vi "GenerateMapGraph.vi"() -> ()   [LabVIEW 2015]
panel:
  out "Numeric 1":i32
  out "Numeric 2":i32
  in  "Graph Parameters":T1={"Y_max"=10.0, "Y_min"=0.0, "X_max"=10.0, "X_min"=0.0}
  out "Output":cluster{dbl[], dbl[]}[](graph)
  in  "Input M":dbl[][](array[numeric])=[[14.0, 12.0, 6.0, 12.0], [10.0, 11.0, 10.0, 10.0], [8.0, 6.0, 10.0, 10.0], [10.0, 9.0, 1.0, 3.0], [0.0, 13.0, 1.0, 7.0]]
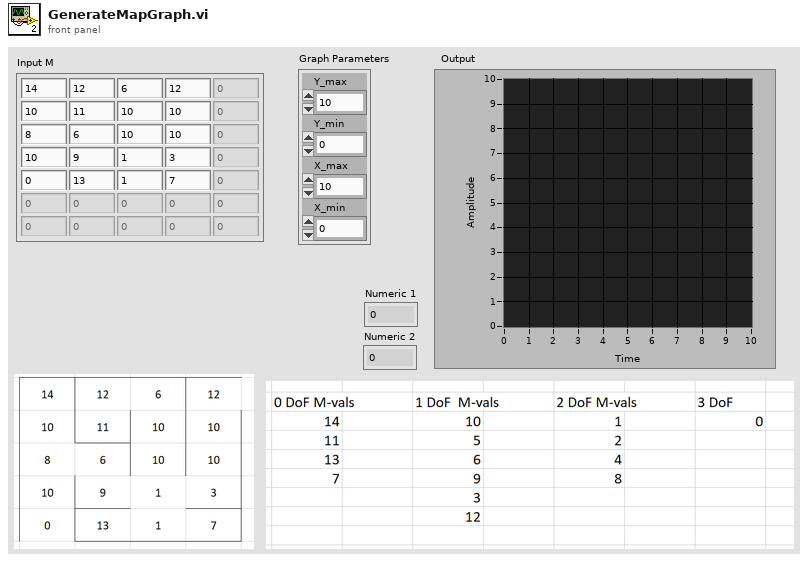
[diagram p1: front panel]
types:
  T1 = cluster{"Y_max":dbl, "Y_min":dbl, "X_max":dbl, "X_min":dbl}
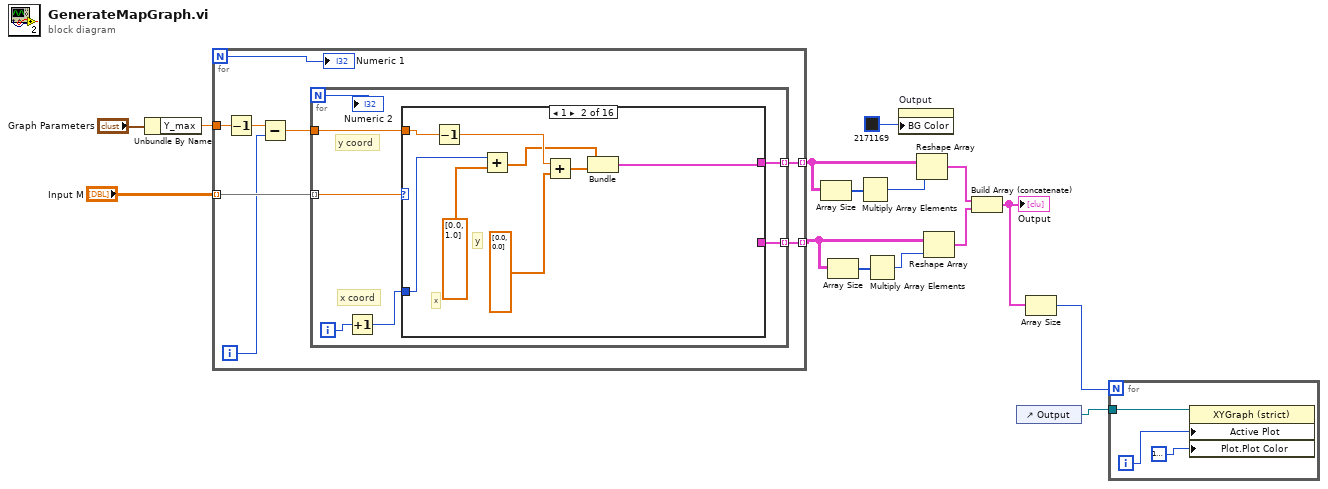
[diagram p0: block diagram]
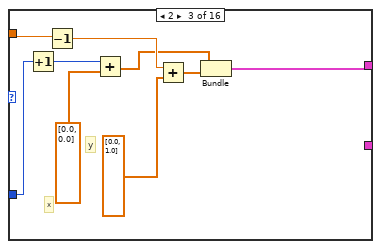
[diagram p3: hidden frame]
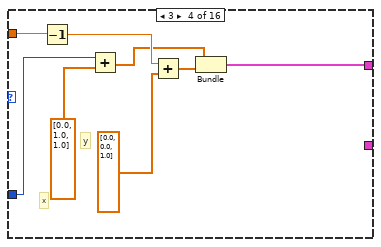
[diagram p4: hidden frame]
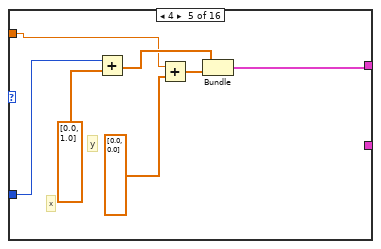
[diagram p5: hidden frame]
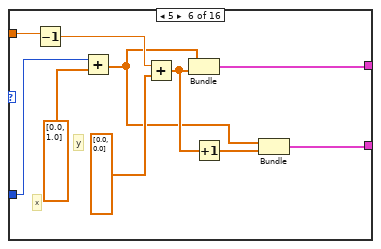
[diagram p6: hidden frame]
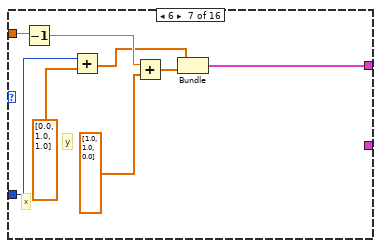
[diagram p7: hidden frame]
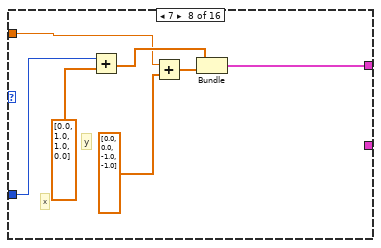
[diagram p8: hidden frame]
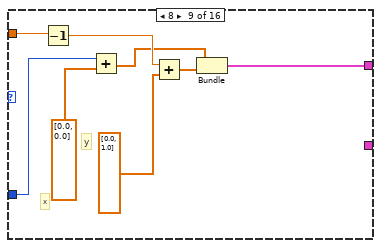
[diagram p9: hidden frame]
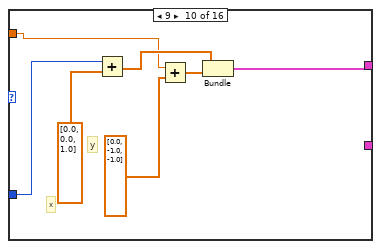
[diagram p10: hidden frame]
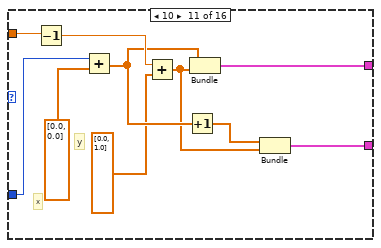
[diagram p11: hidden frame]
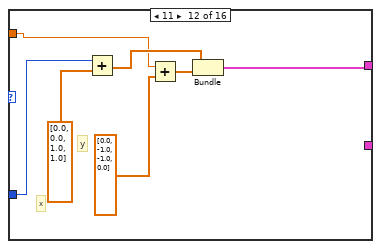
[diagram p12: hidden frame]
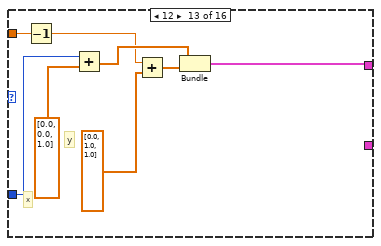
[diagram p13: hidden frame]
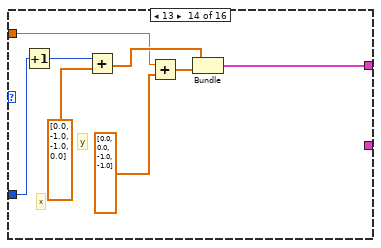
[diagram p14: hidden frame]
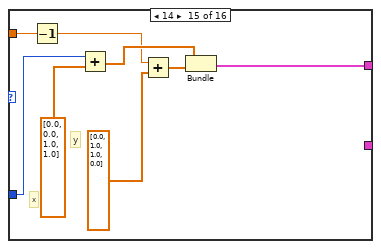
[diagram p15: hidden frame]
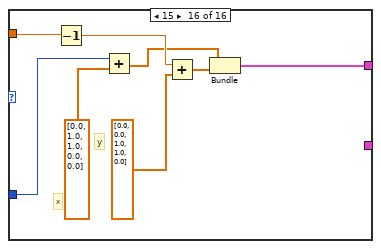
[diagram p16: hidden frame]
diagram:
  n1 = Unbundle By Name("Graph Parameters") -> ("Y_max"=w13:dbl)
  n2 = for {
    N -> [w21]
    tunnel: "Input M" -> [w23] mode=indexing
    tunnel: w13 -> [w22]
    tunnel: [w17] -> w12 mode=indexing
    tunnel: [w16] -> w5 mode=indexing
    i -> [w19]
    n3 = Decrement(x=w22) -> (x-1=w20:dbl)
    n4 = Subtract(x=w20, y=w19) -> (x-y=w18:dbl)
    n5 = for {
      N -> [w29]
      tunnel: w23 -> [w30] mode=indexing
      tunnel: w18 -> [w28]
      tunnel: [w25] -> w17 mode=indexing
      tunnel: [w24] -> w16 mode=indexing
      i -> [w27]
      # "x coord"
      # "y coord"
      n6 = Increment(x=w27) -> (x+1=w26:i32)
      n7 = case shown="1" w30 {
        tunnel: w28 -> [_ w32 w40 w49 w57 w67 w74 w81 w90 w98 w111 w113 w120 w129 w141 w146]
        tunnel: w26 -> [_ w31 w41 w50 w56 w68 w75 w82 w88 w96 w109 w115 w122 w130 w142 w145]
        tunnel: [_ w33 w39 w48 w58 w64 w73 w83 w89 w97 w110 w114 w121 w131 w137 w144] -> w25
        tunnel: [_ _ _ _ _ w63 _ _ _ _ w106 _ _ _ _ _] -> w24
        frame 0, Default {
        }
        frame 1 {
          # "y"
          # "x"
          n8 = Decrement(x=w32) -> (x-1=w38:dbl)
          n9 = Add(x=w31, y=dbl[] [0.0, 1.0] ("appended array")) -> (x+y=w37:dbl[])
          n10 = Add(x=w38, y=dbl[] [0.0, 0.0] ("appended array")) -> (x+y=w36:dbl[])
          n11 = Bundle(w37, w36) -> (w33:cluster{dbl[], dbl[]})  [unwired: 1 in]
        }
        frame 2 {
          # "y"
          # "x"
          n12 = Increment(x=w41) -> (x+1=w42:i32)
          n13 = Decrement(x=w40) -> (x-1=w47:dbl)
          n14 = Add(x=w42, y=dbl[] [0.0, 0.0] ("appended array")) -> (x+y=w46:dbl[])
          n15 = Add(x=w47, y=dbl[] [0.0, 1.0] ("appended array")) -> (x+y=w45:dbl[])
          n16 = Bundle(w46, w45) -> (w39:cluster{dbl[], dbl[]})  [unwired: 1 in]
        }
        frame 3 {
          # "y"
          # "x"
          n17 = Decrement(x=w49) -> (x-1=w55:dbl)
          n18 = Add(x=w50, y=dbl[] [0.0, 1.0, 1.0] ("appended array")) -> (x+y=w54:dbl[])
          n19 = Add(x=w55, y=dbl[] [0.0, 0.0, 1.0] ("appended array")) -> (x+y=w53:dbl[])
          n20 = Bundle(w54, w53) -> (w48:cluster{dbl[], dbl[]})  [unwired: 1 in]
        }
        frame 4 {
          # "y"
          # "x"
          n21 = Add(x=w56, y=dbl[] [0.0, 1.0] ("appended array")) -> (x+y=w62:dbl[])
          n22 = Add(x=w57, y=dbl[] [0.0, 0.0] ("appended array")) -> (x+y=w61:dbl[])
          n23 = Bundle(w62, w61) -> (w58:cluster{dbl[], dbl[]})  [unwired: 1 in]
        }
        frame 5 {
          # "y"
          # "x"
          n24 = Decrement(x=w67) -> (x-1=w69:dbl)
          n25 = Add(x=w68, y=dbl[] [0.0, 1.0] ("appended array")) -> (x+y=w66:dbl[])
          n26 = Add(x=w69, y=dbl[] [0.0, 0.0] ("appended array")) -> (x+y=w72:dbl[])
          n27 = Bundle(w66, w72) -> (w64:cluster{dbl[], dbl[]})  [unwired: 1 in]
          n28 = Increment(x=w72) -> (x+1=w65:dbl[])
          n29 = Bundle(w66, w65) -> (w63:cluster{dbl[], dbl[]})  [unwired: 1 in]
        }
        frame 6 {
          # "y"
          # "x"
          n30 = Decrement(x=w74) -> (x-1=w80:dbl)
          n31 = Add(x=w75, y=dbl[] [0.0, 1.0, 1.0] ("appended array")) -> (x+y=w79:dbl[])
          n32 = Add(x=w80, y=dbl[] [1.0, 1.0, 0.0] ("appended array")) -> (x+y=w78:dbl[])
          n33 = Bundle(w79, w78) -> (w73:cluster{dbl[], dbl[]})  [unwired: 1 in]
        }
        frame 7 {
          # "y"
          # "x"
          n34 = Add(x=w82, y=dbl[] [0.0, 1.0, 1.0, 0.0] ("appended array")) -> (x+y=w87:dbl[])
          n35 = Add(x=w81, y=dbl[] [0.0, 0.0, -1.0, -1.0] ("appended array")) -> (x+y=w86:dbl[])
          n36 = Bundle(w87, w86) -> (w83:cluster{dbl[], dbl[]})  [unwired: 1 in]
        }
        frame 8 {
          # "y"
          # "x"
          n37 = Decrement(x=w90) -> (x-1=w95:dbl)
          n38 = Add(x=w88, y=dbl[] [0.0, 0.0] ("appended array")) -> (x+y=w94:dbl[])
          n39 = Add(x=w95, y=dbl[] [0.0, 1.0] ("appended array")) -> (x+y=w93:dbl[])
          n40 = Bundle(w94, w93) -> (w89:cluster{dbl[], dbl[]})  [unwired: 1 in]
        }
        frame 9 {
          # "y"
          # "x"
          n41 = Add(x=w96, y=dbl[] [0.0, 0.0, 1.0] ("appended array")) -> (x+y=w102:dbl[])
          n42 = Add(x=w98, y=dbl[] [0.0, -1.0, -1.0] ("appended array")) -> (x+y=w101:dbl[])
          n43 = Bundle(w102, w101) -> (w97:cluster{dbl[], dbl[]})  [unwired: 1 in]
        }
        frame 10 {
          # "y"
          # "x"
          n44 = Decrement(x=w111) -> (x-1=w112:dbl)
          n45 = Add(x=w109, y=dbl[] [0.0, 0.0] ("appended array")) -> (x+y=w105:dbl[])
          n46 = Add(x=w112, y=dbl[] [0.0, 1.0] ("appended array")) -> (x+y=w103:dbl[])
          n47 = Increment(x=w105) -> (x+1=w107:dbl[])
          n48 = Bundle(w105, w103) -> (w110:cluster{dbl[], dbl[]})  [unwired: 1 in]
          n49 = Bundle(w107, w103) -> (w106:cluster{dbl[], dbl[]})  [unwired: 1 in]
        }
        frame 11 {
          # "y"
          # "x"
          n50 = Add(x=w115, y=dbl[] [0.0, 0.0, 1.0, 1.0] ("appended array")) -> (x+y=w116:dbl[])
          n51 = Add(x=w113, y=dbl[] [0.0, -1.0, -1.0, 0.0] ("appended array")) -> (x+y=w117:dbl[])
          n52 = Bundle(w116, w117) -> (w114:cluster{dbl[], dbl[]})  [unwired: 1 in]
        }
        frame 12 {
          # "y"
          # "x"
          n53 = Decrement(x=w120) -> (x-1=w123:dbl)
          n54 = Add(x=w122, y=dbl[] [0.0, 0.0, 1.0] ("appended array")) -> (x+y=w124:dbl[])
          n55 = Add(x=w123, y=dbl[] [0.0, 1.0, 1.0] ("appended array")) -> (x+y=w125:dbl[])
          n56 = Bundle(w124, w125) -> (w121:cluster{dbl[], dbl[]})  [unwired: 1 in]
        }
        frame 13 {
          # "y"
          # "x"
          n57 = Increment(x=w130) -> (x+1=w128:i32)
          n58 = Add(x=w128, y=dbl[] [0.0, -1.0, -1.0, 0.0] ("appended array")) -> (x+y=w135:dbl[])
          n59 = Add(x=w129, y=dbl[] [0.0, 0.0, -1.0, -1.0] ("appended array")) -> (x+y=w134:dbl[])
          n60 = Bundle(w135, w134) -> (w131:cluster{dbl[], dbl[]})  [unwired: 1 in]
        }
        frame 14 {
          # "y"
          # "x"
          n61 = Decrement(x=w141) -> (x-1=w136:dbl)
          n62 = Add(x=w142, y=dbl[] [0.0, 0.0, 1.0, 1.0] ("appended array")) -> (x+y=w138:dbl[])
          n63 = Add(x=w136, y=dbl[] [0.0, 1.0, 1.0, 0.0] ("appended array")) -> (x+y=w139:dbl[])
          n64 = Bundle(w138, w139) -> (w137:cluster{dbl[], dbl[]})  [unwired: 1 in]
        }
        frame 15 {
          # "y"
          # "x"
          n65 = Decrement(x=w146) -> (x-1=w151:dbl)
          n66 = Add(x=w145, y=dbl[] [0.0, 1.0, 1.0, 0.0, 0.0] ("appended array")) -> (x+y=w150:dbl[])
          n67 = Add(x=w151, y=dbl[] [0.0, 0.0, 1.0, 1.0, 0.0] ("appended array")) -> (x+y=w149:dbl[])
          n68 = Bundle(w150, w149) -> (w144:cluster{dbl[], dbl[]})  [unwired: 1 in]
        }
      }
      "Numeric 2" <- w29
    }
    "Numeric 1" <- w21
  }
  n69 = Array Size(array=w12) -> (size(s)=w11:i32[])
  n70 = Array Size(array=w5) -> (size(s)=w6:i32[])
  n71 = Multiply Array Elements(1:w11) -> (0:w8:i32)
  n72 = Multiply Array Elements(1:w6) -> (0:w7:i32)
  n73 = property on="Output" class="XYGraph (strict)"("BG Color"=u32 2171169) -> ()  [unwired: 2 in, 2 out]
  n74 = Reshape Array(w12, w8) -> (w4:cluster{dbl[], dbl[]}[])
  n75 = Reshape Array(w5, w7) -> (w3:cluster{dbl[], dbl[]}[])
  n76 = Build Array (concatenate)(w4, w3) -> (w2:cluster{dbl[], dbl[]}[])
  "Output" <- w2
  n77 = control-ref of="Output"() -> (w9:refnum<vi>)
  n78 = Array Size(array=w2) -> (size(s)=w1:i32)
  n79 = for {
    N: w1 -> [_]
    tunnel: w9 -> [w154]
    i -> [w152]
    n80 = property class="XYGraph (strict)"(reference=w154, "Active Plot"=w152, "Plot.Plot Color"=u32 16777226) -> ()  [unwired: 1 in, 2 out]
  }
